vi "Get Device Property.vi"   [LabVIEW 2020, in "SLSC.lvlib"]
doc: "Gets the value of the specified device property from one or more devices. You can use an array instance of this VI to get a scalar property from multiple devices with a single call to the VI."
uses:
  <vilib>/SLSC/SLSC.lvlib
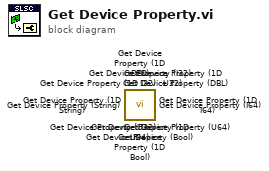
[diagram p0: block diagram]
diagram:
  n1 = call <vilib>:"Get Device Property (1D U64).vi"() -> ()  [unwired: 13 in, 3 out]
  n2 = call <vilib>:"Get Device Property (1D U32).vi"() -> ()  [unwired: 13 in, 3 out]
  n3 = call <vilib>:"Get Device Property (1D String).vi"() -> ()  [unwired: 13 in, 3 out]
  n4 = call <vilib>:"Get Device Property (1D I64).vi"() -> ()  [unwired: 13 in, 3 out]
  n5 = call <vilib>:"Get Device Property (1D I32).vi"() -> ()  [unwired: 13 in, 3 out]
  n6 = call <vilib>:"Get Device Property (1D DBL).vi"() -> ()  [unwired: 13 in, 3 out]
  n7 = call <vilib>:"Get Device Property (1D Bool).vi"() -> ()  [unwired: 13 in, 3 out]
  n8 = call <vilib>:"Get Device Property (U64).vi"() -> ()  [unwired: 13 in, 3 out]
  n9 = call <vilib>:"Get Device Property (U32).vi"() -> ()  [unwired: 13 in, 3 out]
  n10 = call <vilib>:"Get Device Property (String).vi"() -> ()  [unwired: 13 in, 3 out]
  n11 = call <vilib>:"Get Device Property (I64).vi"() -> ()  [unwired: 13 in, 3 out]
  n12 = call <vilib>:"Get Device Property (I32).vi"() -> ()  [unwired: 13 in, 3 out]
  n13 = call <vilib>:"Get Device Property (DBL).vi"() -> ()  [unwired: 13 in, 3 out]
  n14 = call <vilib>:"Get Device Property (Bool).vi"() -> ()  [unwired: 13 in, 3 out]
